vi "DAC Run.vi"(8 "error in":errorcluster, 11 "DAC ADV in":refnum<class "DAC ADV.lvclass">) -> (0 "error out":errorcluster, 3 "DAC ADV out":refnum<class "DAC ADV.lvclass">)   [LabVIEW 2019, in "DAC.lvlib" / "DAC ADV.lvclass"]
uses:
  DAC ADV.lvclass
  C:/Users/wg/Documents/LV_Projects/test-stand/App/DAC/DAC.lvclass
  DAC.lvclass/DAC.ctl
  Results/Results Method.ctl
  Results/Water Tunnel Results/Water Tunnel Results.lvclass
  DAC ADV.lvclass/DAC ADV.ctl
  DAC.lvclass
  Results/Results.lvlib
panel:
  out "read buffer":string
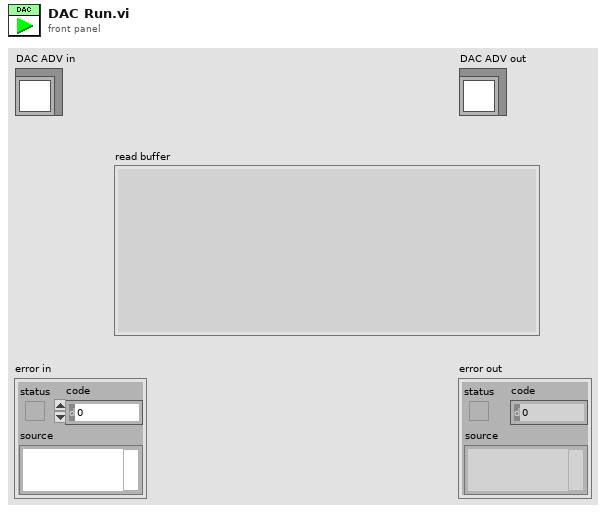
[diagram p1: front panel]
types:
  T1 = typedef "Results.lvlib/Results Method.ctl" = enum16{"Get", "Set"}
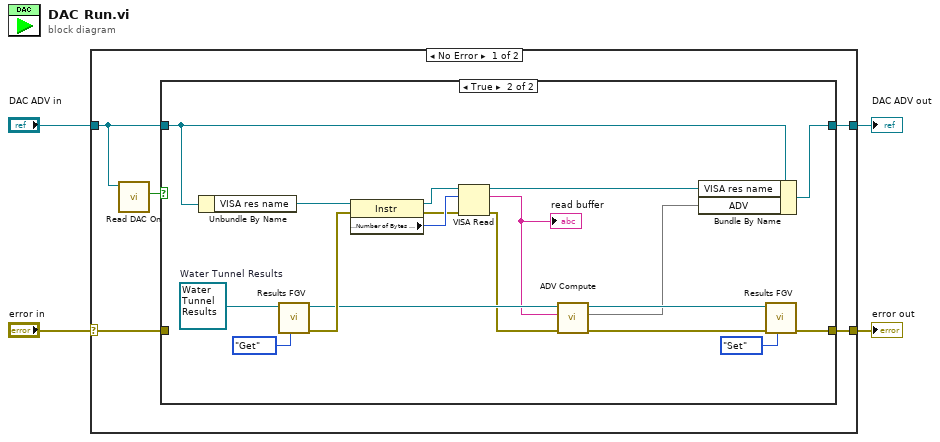
[diagram p0: block diagram]
diagram:
  n1 = case shown="No Error" "error in" {
    selector: "error in" -> [w7 w31]
    tunnel: [w6 w31] -> w2
    tunnel: [w8 w30] -> w1
    tunnel: "DAC ADV in" -> [w5 w30]
    frame No Error {
      n2 = call "Read DAC On.vi"("DAC in"=w5) -> ("DAC On"=w9:bool)  [unwired: 8 in, 2 out]
      n3 = case shown="True" w9 {
        tunnel: w5 -> [w11 w29]
        tunnel: [w11 w26] -> w8
        tunnel: w7 -> [w10 _]
        tunnel: [w10 w25] -> w6
        frame False {
        }
        frame True {
          w24 = refnum<class "Water Tunnel Results.lvclass"> refnum  # Water Tunnel Results
          n4 = Unbundle By Name(w29) -> ("VISA res name"=w23:refnum<visa-resource-name>)
          n5 = call-dynamic "Results FGV.vi"("Method"=Results_Method."Get", "Water Tunnel Results in"=w24) -> ("error out"=w22:errorcluster, "Water Tunnel  Results out"=w17:refnum<class "Water Tunnel Results.lvclass">)  [unwired: 8 in]
          n6 = property class="Instr"(reference=w23, error in=w22) -> (reference out=w21:refnum<visa-resource-name>, error out=w19:errorcluster, "Serial Settings:Number of Bytes at Serial Port"=w20:u32)
          n7 = VISA Read(VISA resource name=w21, byte count=w20, error in (no error)=w19) -> (VISA resource name out=w18:refnum<visa-resource-name>, read buffer=w13:string, error out=w15:errorcluster)  [unwired: 1 out]
          "read buffer" <- w13
          n8 = call "ADV Compute.vi"("error in"=w15, "ADV String"=w13, "Water Tunnel Results in"=w17) -> ("error out"=w14:errorcluster, 2:w12, "Water Tunnel Results out"=w16:refnum<class "Water Tunnel Results.lvclass">)  [unwired: 6 in]
          n9 = Bundle By Name(cluster=w29, "VISA res name"=w18, "ADV"=w12) -> (w26:refnum<class "DAC ADV.lvclass">)
          n10 = call-dynamic "Results FGV.vi"("Method"=Results_Method."Set", "error in"=w14, "Water Tunnel Results in"=w16) -> ("error out"=w25:errorcluster)  [unwired: 7 in, 1 out]
        }
      }
    }
    frame Error {
    }
  }
  "error out" <- w2
  "DAC ADV out" <- w1
